vi "niRFUtil MEAS Peak Search.vi"(0 "Waveform In":T1 {"y" min=0 max=127 format="%.2f"; "dx" format="%^.2e"; "x0" format="%^.2e"}, 5 "Peak Threshold Enabled":T4=enum."True", 7 "Peak Threshold(dBm)":dbl=-90.0 format="%.2g", 9 "Peak Excursion Enabled":T3, 11 "Peak Excursion (dB)":dbl=6.0 format="%.2g", 12 "Chunk Size":i32=32768) -> (4 "Peak Indices":i32[](array[numeric]), 6 "Peak Amplitudes":sgl[](array[numeric]), 8 "Number of Peaks":i32)   [LabVIEW 2015, in "niRFUtil.lvlib"]
uses:
  niRFUtil.lvlib
  Includes/niRFUtil INC Peak Threshold Enabled.ctl
  Includes/niRFUtil INC Peak Excursion Enabled.ctl
  Includes/niRFUtil INC Real Waveform.ctl
  Includes/niRFUtil INC Real Array.ctl
  <vilib>/Analysis/NI_AAL_SigProc.lvlib
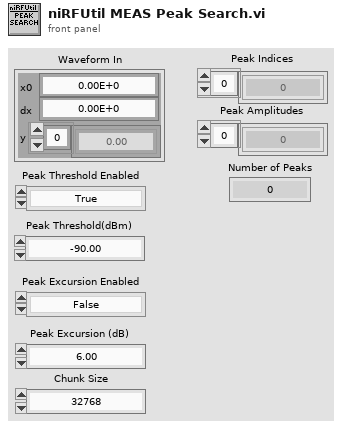
[diagram p1: front panel]
types:
  T1 = typedef "niRFUtil.lvlib/niRFUtil INC Real Waveform.ctl" = cluster{"x0":dbl, "dx":dbl, "y":T2}
  T2 = typedef "niRFUtil.lvlib/niRFUtil INC Real Array.ctl" = sgl[]
  T3 = typedef "niRFUtil.lvlib/niRFUtil INC Peak Excursion Enabled.ctl" = enum16{"False", "True"}
  T4 = typedef "niRFUtil.lvlib/niRFUtil INC Peak Threshold Enabled.ctl" = enum16{"False", "True"}
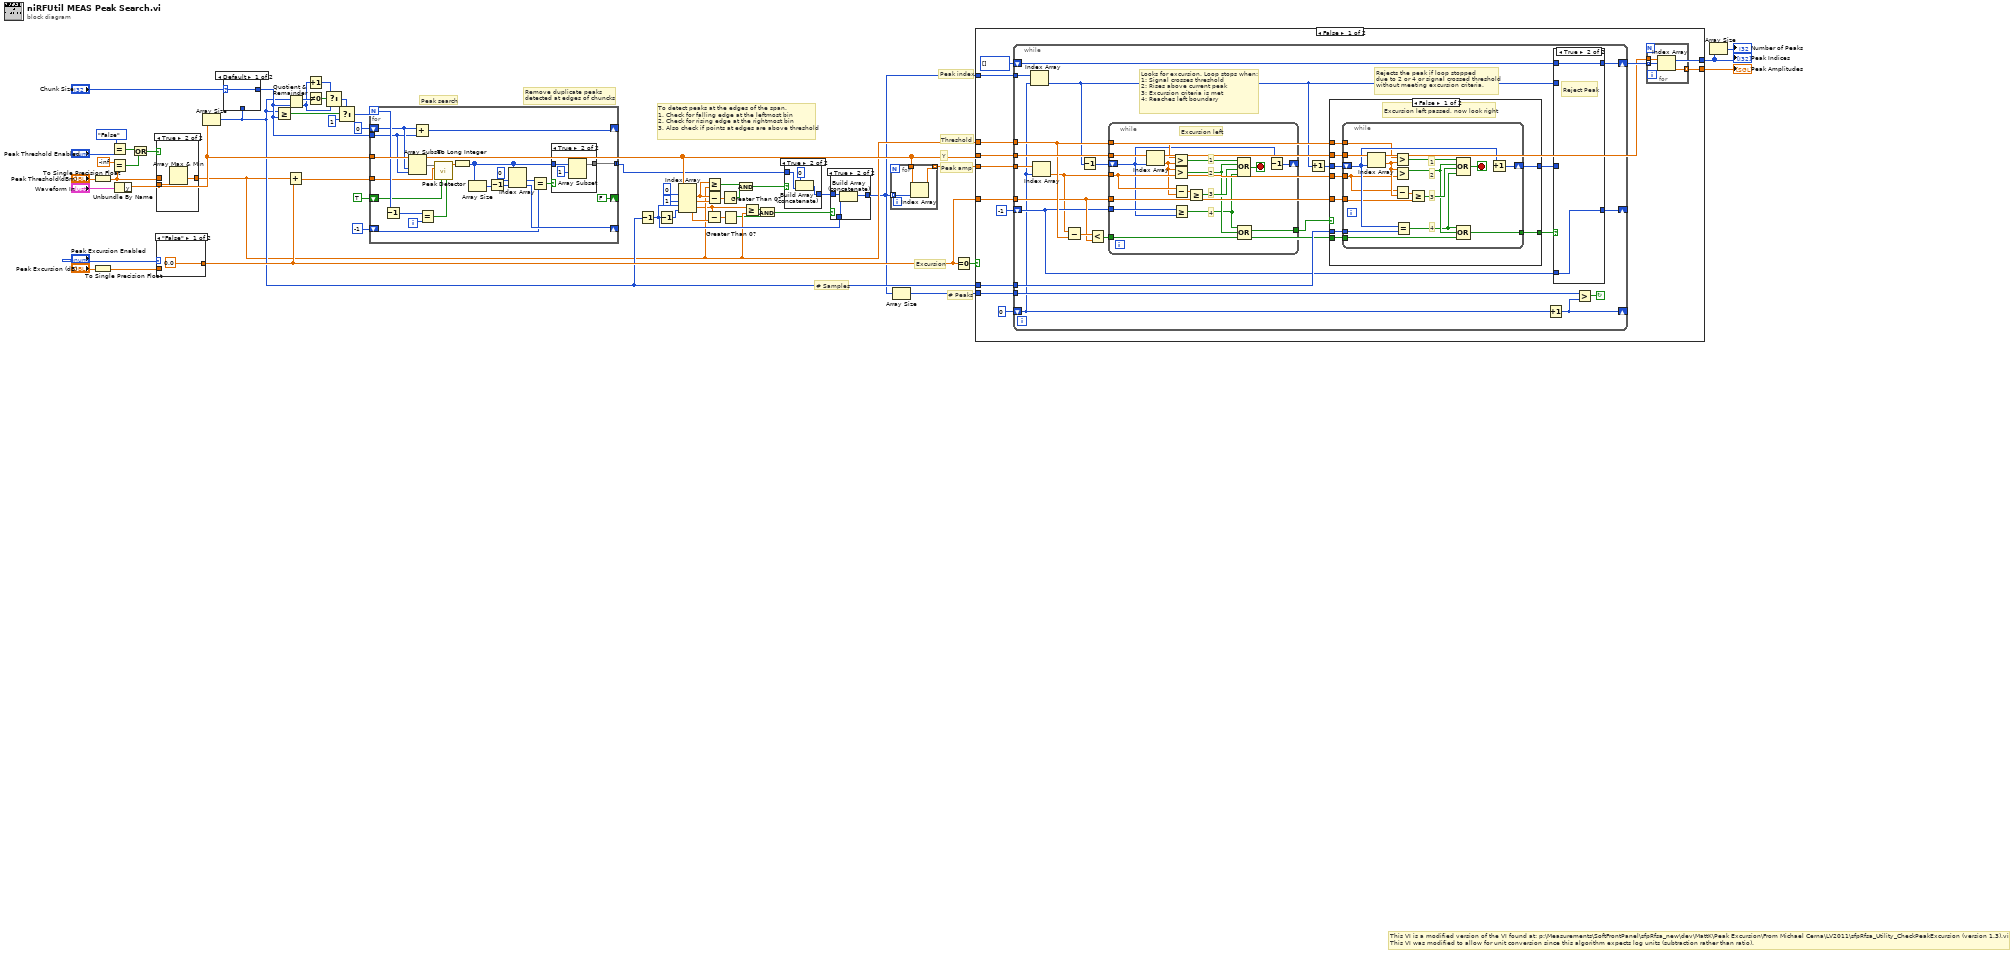
[diagram p0: block diagram]
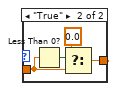
[diagram p5: hidden frame]
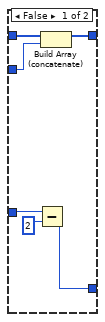
[diagram p8: hidden frame]
diagram:
  # "Peak search"
  # "Remove duplicate peaks\ndetected at edges of chuncks"
  # "Y"
  # "Peak amp"
  # "Threshold"
  # "Excursion"
  # "To detect peaks at the edges of the span. \n1. Check for falling edge at the leftmost bin\n2. Check for rising edge at the rightmost bin\n3. Also check if points at edges are above threshold"
  # "# Samples"
  # "# Peaks"
  # "Peak index"
  # "This VI is a modified version of the VI found at: p:\\Measurements\\SoftFrontPanel\\sfpRfsa_new\\dev\\MattK\\Peak Excursion\\From Michael Cerna\\LV2011\\sfpRfsa_Utility_CheckPeakExcursion (version 1.3).vi \nThis VI was modified to allow for unit conversion since this algorithm expects log units (subtraction rather than ratio)."
  n1 = To Single Precision Float(number="Peak Threshold(dBm)") -> (single precision float=w2:sgl)
  n2 = To Single Precision Float(number="Peak Excursion (dB)") -> (single precision float=w6:sgl)
  n3 = Equal?(x=niRFUtil_INC_Peak_Threshold_Enabled."False" ("Peak Threshold Enabled"), y="Peak Threshold Enabled") -> (x = y?=w13:bool)
  n4 = Equal?(x=sgl -inf, y=w2) -> (x = y?=w12:bool)
  n5 = Unbundle By Name("Waveform In") -> ("y"=w31:T2)
  n6 = Or(x=w13, y=w12) -> (x .or. y?=w11:bool)
  n7 = case shown="True" w11 {
    tunnel: w31 -> [_ w58]
    tunnel: [w56 w57] -> w22
    tunnel: w2 -> [w56 _]
    frame False {
    }
    frame True {
      n8 = Array Max & Min(array=w58) -> (min value=w57:sgl)  [unwired: 3 out]
    }
  }
  n9 = case shown="\"False\"" "Peak Excursion Enabled" {
    tunnel: [sgl 0.0 ("upper limit") w63] -> w35
    tunnel: w6 -> [_ w60]
    frame "False" {
    }
    frame "True" {
      n10 = Less Than 0?(x=w60) -> (x < 0?=w62:bool)
      n11 = Select(t=sgl 0.0, s=w62, f=w60) -> (s? t:f=w63:sgl)
    }
  }
  n12 = Array Size(array=w31) -> (size(s)=w26:i32)
  n13 = case shown="Default" "Chunk Size" {
    selector: "Chunk Size" -> [w64 _]
    tunnel: [w64 w65] -> w28
    tunnel: w26 -> [_ w65]
    frame Default {
    }
    frame -1 {
    }
  }
  n14 = Greater Or Equal?(x=w26, y=w28) -> (x >= y?=w51:bool)
  n15 = Add(x=w22, y=w35) -> (x+y=w45:sgl)
  n16 = Quotient & Remainder(x=w26, y=w28) -> (x-y*floor(x/y)=w54:i32, floor(x/y)=w4:i32)
  n17 = Increment(x=w4) -> (x+1=w3:i32)
  n18 = Not Equal To 0?(x=w54) -> (x != 0?=w53:bool)
  n19 = Select(t=w3, s=w53, f=w4) -> (s? t:f=w52:i32)
  n20 = Select(t=w52, s=w51, f=1) -> (s? t:f=w49:i32)
  n21 = for {
    N: w49 -> [w86]
    tunnel: w31 -> [w87]
    tunnel: w45 -> [w83]
    tunnel: w28 -> [w67]
    shift-right: [FALSE] -> _
    shift-left: TRUE -> [w81]
    tunnel: [w75] -> w17 mode=concatenating
    shift-right: [w72] -> _
    shift-left: -1 -> [w70]
    shift-right: [w66] -> _
    shift-left: 0 ("f") -> [w68]
    i -> [w74]
    n22 = Decrement(x=w86) -> (x-1=w85:i32)
    n23 = Array Subset(array=w87, index=w68, length=w67) -> (w84:T2)
    n24 = Add(x=w68, y=w67) -> (x+y=w66:i32)
    n25 = Equal?(x=w85, y=w74) -> (x = y?=w80:bool)
    n26 = call <vilib>:"Peak Detector.vi"("end of data (T)"=w80, "initialize (T)"=w81, "threshold"=w83, "X"=w84) -> ("Locations"=w79:dbl[])  [unwired: 3 in, 4 out]
    n27 = To Long Integer(number=w79) -> (32bit integer=w76:i32[])
    n28 = Array Size(array=w76) -> (size(s)=w77:i32)
    n29 = Decrement(x=w77) -> (x-1=w73:i32)
    n30 = Index Array(array=w76, index #1=0 ("index"), index #2=w73) -> (element #1=w71:i32, element #2=w72:i32)
    n31 = Equal?(x=w71, y=w70) -> (x = y?=w69:bool)
    n32 = case shown="True" w69 {
      tunnel: w76 -> [w88 w91]
      tunnel: [w88 w89] -> w75
      frame False {
      }
      frame True {
        n33 = Array Subset(array=w91, index=1) -> (w89:i32[])  [unwired: 1 in]
      }
    }
  }
  n34 = Decrement(x=w26) -> (x-1=w37:i32)
  n35 = Decrement(x=w37) -> (x-1=w42:i32)
  n36 = Index Array(array=w31, index #1=0 ("index"), index #2=1 ("index"), index #3=w37, index #4=w42) -> (element #1=w24:sgl, element #2=w41:sgl, element #3=w19:sgl, element #4=w40:sgl)
  n37 = Subtract(x=w19, y=w40) -> (x-y=w38:sgl)
  n38 = Greater Or Equal?(x=w24, y=w22) -> (x >= y?=w23:bool)
  n39 = Subtract(x=w24, y=w41) -> (x-y=w39:sgl)
  n40 = Greater Than 0?(x=w39) -> (x > 0?=w25:bool)
  n41 = Greater Than 0?(x=w38) -> (x > 0?=w21:bool)
  n42 = And(x=w23, y=w25) -> (x .and. y?=w18:bool)
  n43 = Greater Or Equal?(x=w19, y=w22) -> (x >= y?=w20:bool)
  n44 = And(x=w20, y=w21) -> (x .and. y?=w16:bool)
  n45 = case shown="True" w18 {
    tunnel: w17 -> [w92 w94]
    tunnel: [w92 w95] -> w15
    frame False {
    }
    frame True {
      n46 = Build Array (concatenate)(0 ("index"), w94) -> (w95:i32[])
    }
  }
  n47 = case shown="True" w16 {
    tunnel: w15 -> [w96 w99]
    tunnel: w37 -> [_ w98]
    tunnel: [w96 w97] -> w14
    frame False {
    }
    frame True {
      n48 = Build Array (concatenate)(w99, w98) -> (w97:i32[])
    }
  }
  n49 = for {
    tunnel: w31 -> [w102]
    tunnel: w14 -> [w101] mode=indexing
    tunnel: [w100] -> w47 mode=indexing
    n50 = Index Array(array=w102, index=w101) -> (element=w100:sgl)
  }
  n51 = Array Size(array=w14) -> (size(s)=w46:i32)
  n52 = Equal To 0?(x=w35) -> (x = 0?=w55:bool)
  n53 = case shown="False" w55 {
    tunnel: [w105 w193] -> w32
    tunnel: w35 -> [w114 _]
    tunnel: w22 -> [w112 _]
    tunnel: w47 -> [w110 w192]
    tunnel: w14 -> [w107 w193]
    tunnel: w46 -> [w109 _]
    tunnel: w31 -> [w104 _]
    tunnel: w26 -> [w106 _]
    tunnel: [w103 w192] -> w34
    frame False {
      n54 = while {
        tunnel: w107 -> [w124]
        tunnel: w114 -> [w132]
        shift-right: [w138] -> w105
        shift-left: i32[] [] -> [w140]
        tunnel: w104 -> [w130]
        shift-right: [w122] -> _
        shift-left: 0 -> [w118]
        tunnel: w110 -> [w123]
        tunnel: w112 -> [w134]
        tunnel: w106 -> [w135]
        shift-right: [w128] -> _
        shift-left: -1 -> [w129]
        tunnel: w109 -> [w125]
        stop <- w136 continue-if-true
        # "Rejects the peak if loop stopped\ndue to 2 or 4 or signal crossed threshold\nwithout meeting excursion criteria."
        # "Looks for excursion. Loop stops when:\n1: Signal crosses threshold\n2: Rises above current peak\n3: Excursion criteria is met\n4: Reaches left boundary"
        n55 = Index Array(array=w124, index=w118) -> (element=w120:i32)
        n56 = Index Array(array=w123, index=w118) -> (element=w126:sgl)
        n57 = Subtract(x=w126, y=w134) -> (x-y=w133:sgl)
        n58 = Decrement(x=w120) -> (x-1=w121:i32)
        n59 = Less?(x=w133, y=w132) -> (x < y?=w131:bool)
        n60 = while {
          tunnel: w130 -> [w191]
          shift-right: [w186] -> _
          shift-left: w121 -> [w177]
          tunnel: w126 -> [w183]
          tunnel: w132 -> [w181]
          tunnel: w129 -> [w178]
          tunnel: [w188] -> w127
          tunnel: w134 -> [w182]
          tunnel: w131 -> [w179]
          stop <- w189 stop-if-true
          # "Excursion left"
          # "3"
          # "4"
          # "2"
          # "1"
          n61 = Index Array(array=w191, index=w177) -> (element=w180:sgl)
          n62 = Greater?(x=w182, y=w180) -> (0:w184:bool)
          n63 = Greater?(x=w180, y=w183) -> (0:w185:bool)
          n64 = Subtract(x=w183, y=w180) -> (x-y=w190:sgl)
          n65 = Greater Or Equal?(x=w178, y=w177) -> (x >= y?=w176:bool)
          n66 = Greater Or Equal?(x=w190, y=w181) -> (x >= y?=w187:bool)
          n67 = Compound Arithmetic op=OR(w184, w185, w187, w176) -> (w189:bool)
          n68 = Compound Arithmetic op=OR(w176, w185, w179) -> (w188:bool)
          n69 = Decrement(x=w177) -> (x-1=w186:i32)
        }
        n70 = Increment(x=w120) -> (x+1=w119:i32)
        n71 = case shown="False" w127 {
          selector: w127 -> [_ w175]
          tunnel: w130 -> [w157 _]
          tunnel: w132 -> [w156 _]
          tunnel: w126 -> [w152 _]
          tunnel: [w155 w175] -> w139
          tunnel: w119 -> [w154 w174]
          tunnel: w135 -> [w153 _]
          tunnel: [w151 w174] -> w137
          tunnel: w134 -> [w150 _]
          tunnel: w131 -> [w149 _]
          frame False {
            # "Excursion left passed, now look right"
            n72 = while {
              tunnel: w157 -> [w173]
              shift-right: [w166] -> w151
              shift-left: w154 -> [w167]
              tunnel: w152 -> [w162]
              tunnel: w156 -> [w161]
              tunnel: w153 -> [w169]
              tunnel: [w168] -> w155
              tunnel: w150 -> [w163]
              tunnel: w149 -> [w158]
              stop <- w170 stop-if-true
              # "4"
              # "3"
              # "2"
              # "1"
              n73 = Index Array(array=w173, index=w167) -> (element=w164:sgl)
              n74 = Greater?(x=w163, y=w164) -> (0:w160:bool)
              n75 = Greater?(x=w164, y=w162) -> (0:w165:bool)
              n76 = Subtract(x=w162, y=w164) -> (x-y=w172:sgl)
              n77 = Equal?(x=w167, y=w169) -> (x = y?=w159:bool)
              n78 = Greater Or Equal?(x=w172, y=w161) -> (x >= y?=w171:bool)
              n79 = Compound Arithmetic op=OR(w160, w165, w171, w159) -> (w170:bool)
              n80 = Compound Arithmetic op=OR(w159, w165, w158) -> (w168:bool)
              n81 = Increment(x=w167) -> (x+1=w166:i32)
            }
          }
          frame True {
            # "excursion left failed - peak rejected"
          }
        }
        n82 = Increment(x=w118) -> (x+1=w122:i32)
        n83 = case shown="True" w139 {
          tunnel: w140 -> [w146 w148]
          tunnel: [w145 w148] -> w138
          tunnel: w137 -> [w143 _]
          tunnel: [w141 w147] -> w128
          tunnel: w129 -> [_ w147]
          tunnel: w120 -> [w144 _]
          frame False {
            n84 = Subtract(x=w143, y=2) -> (x-y=w141:i32)
            n85 = Build Array (concatenate)(w146, w144) -> (w145:i32[])
          }
          frame True {
            # "Reject Peak"
          }
        }
        n86 = Greater?(x=w125, y=w122) -> (0:w136:bool)
      }
      n87 = for {
        tunnel: [w117] -> w103 mode=indexing
        tunnel: w105 -> [w116] mode=indexing
        tunnel: w104 -> [w115]
        n88 = Index Array(array=w115, index=w116) -> (element=w117:sgl)
      }
    }
    frame True {
    }
  }
  "Peak Amplitudes" <- w34
  "Peak Indices" <- w32
  n89 = Array Size(array=w32) -> (size(s)=→"Number of Peaks":i32)
